vi "VI tree.vi"   [LabVIEW 2021]
panel:
  # "VI tree in diagram"
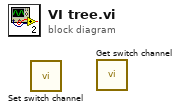
[diagram p0: block diagram]
diagram:
  n1 = call "Set switch channel.vi"() -> ()  [unwired: 10 in, 2 out]
  n2 = call "Get switch channel.vi"() -> ()  [unwired: 9 in, 3 out]
